vi "Automation_TaskFailed.vi"(8 "error in (no error)":errorcluster, 9 "device error":errorcluster, 10 "Correlation ID":u32, 11 "Application in":refnum<class "Application.lvclass">) -> (0 "error out":errorcluster, 3 "Application out":refnum<class "Application.lvclass">)   [LabVIEW 2023, in "Application.lvlib" / "Application.lvclass"]
uses:
  Application.lvclass
  Application.lvclass/Application.ctl
  Automation/AutomationContext.lvclass
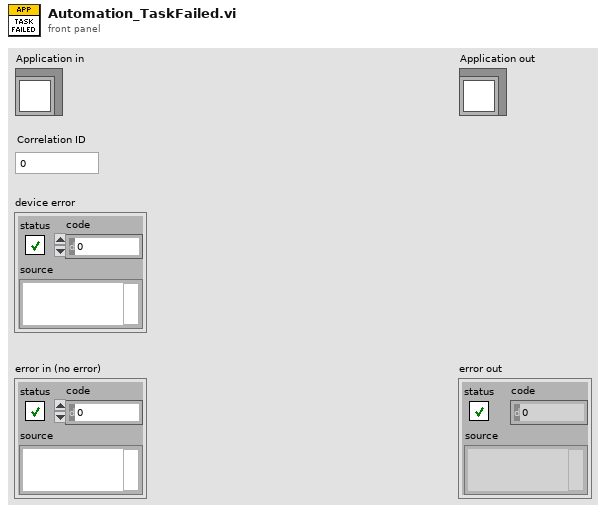
[diagram p1: front panel]
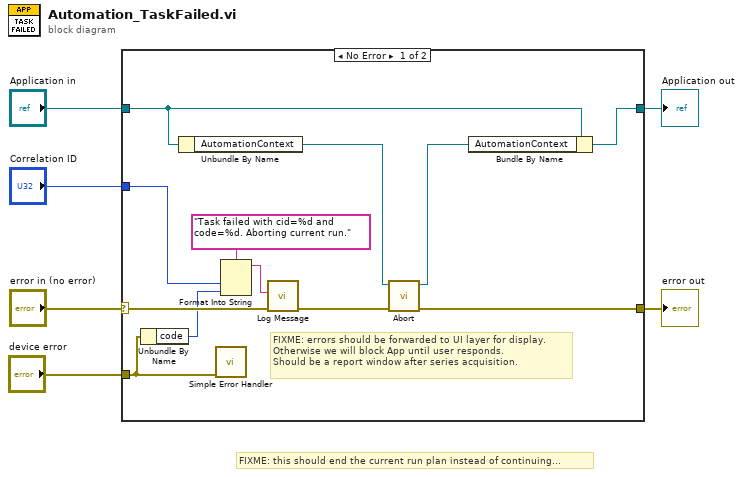
[diagram p0: block diagram]
diagram:
  # "FIXME: this should end the current run plan instead of continuing..."
  n1 = case shown="No Error" "error in (no error)" {
    selector: "error in (no error)" -> [w16 w20]
    tunnel: [w7 w20] -> w5
    tunnel: [w17 w19] -> w3
    tunnel: "Application in" -> [w18 w19]
    tunnel: "Correlation ID" -> [w14 _]
    tunnel: "device error" -> [w11 _]
    frame No Error {
      # "FIXME: errors should be forwarded to UI layer for display.\nOtherwise we will block App until user responds.\nShould be a report window after series acquisition."
      n2 = Unbundle By Name(w11) -> ("code"=w12:i32)
      n3 = Unbundle By Name(w18) -> ("AutomationContext"=w10:refnum<class "AutomationContext.lvclass">)
      n4 = call <vilib>:"Simple Error Handler.vi"("error in (no error)"=w11) -> ()  [unwired: 4 in, 5 out]
      n5 = Format Into String(format string="Task failed with cid=%d and code=%d. Aborting current run.", w14, w12) -> (resulting string=w15:string)  [unwired: 2 in, 1 out]
      n6 = call "Log Message.vi"("error constant"=w16, "input"=w15) -> ("error constant 2"=w8:errorcluster)  [unwired: 8 in, 1 out]
      n7 = call "Abort.vi"("error in (no error)"=w8, "AutomationContext in"=w10) -> ("error out"=w7:errorcluster, "AutomationContext out"=w9:refnum<class "AutomationContext.lvclass">)  [unwired: 8 in]
      n8 = Bundle By Name(cluster=w18, "AutomationContext"=w9) -> (w17:refnum<class "Application.lvclass">)
    }
    frame Error {
    }
  }
  "error out" <- w5
  "Application out" <- w3
